vi "Pre Launch Init.vi"(11 "CameraTestingUI in":refnum<class "CameraTestingENI.lvclass">) -> (0 "error out":errorcluster, 3 "CameraTestingUI out":refnum<class "CameraTestingENI.lvclass">)   [LabVIEW 2020, in "CameraTestingProxy.lvlib" / "CameraTestingENI.lvclass"]
doc: "(<B>Filename</B>: Actor Framework.lvlib:Actor.lvclass:Pre Launch Init.vi)\n\nDefines behavior that occurs after the Launch Nested Actor method is invoked but before the actor's Actor Core method begins running.\n\nBy default, this method does nothing. A descendant class may override it to define behavior."
uses:
  CameraTestingENI.lvclass
  Private/TypeDef/PreLaunchInitState.ctl
  CameraTestingENI.lvclass/CameraTestingENI.ctl
  CameraTestingApp/ICameraTesting/ICameraTesting/TypeDef/Events.ctl
  Camera/ICamera/ICamera/TypeDef/SnapInfo.ctl
  CameraTestingApp/ICameraTesting/ICameraTesting/TypeDef/FrameRateValReceived.ctl
  CameraTestingApp/ICameraTesting/ICameraTesting/TypeDef/ImgTypeValReceived.ctl
  CameraTestingApp/ICameraTesting/ICameraTesting/TypeDef/ResolutionValReceived.ctl
  CameraTestingApp/ICameraTesting/ICameraTesting/TypeDef/VideoOptCodesUpdated.ctl
  CameraTestingApp/ICameraTesting/ICameraTesting/TypeDef/VideoOptionsInfo.ctl
  CameraTestingApp/ICameraTesting/ICameraTesting/TypeDef/StatusUpdated.ctl
  CameraTestingApp/ICameraTesting/ICameraTesting/TypeDef/StatusRecord.ctl
  CameraTestingApp/ICameraTesting/ICameraTesting/TypeDef/VideoBufferUpdate.ctl
  Private/TypeDef/CamTestEnqrReceived.ctl
  Private/TypeDef/QuitActorEvn.ctl
  Private/TypeDef/HelperLoopCamTestEvn.ctl
  Private/TypeDef/VideoLoopCamTestEvn.ctl
  <vilib>/ActorFramework/Actor/Actor.lvclass
  Camera/ICamera/ICamera/ICamera.lvclass
  CameraTestingApp/ICameraTesting/ICameraTesting/ICameraTesting.lvclass
  <vilib>/ActorFramework/Message Enqueuer/Message Enqueuer.lvclass
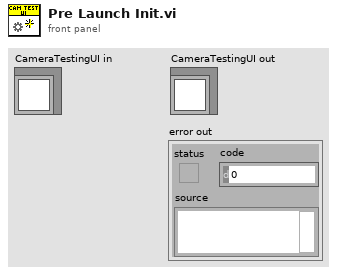
[diagram p1: front panel]
types:
  T1 = typedef "CameraTestingProxy.lvlib/CameraTestingENI.lvclass/PreLaunchInitState.ctl" = enum16{"Create Events", "Registration Events"}
  T2 = typedef "CameraTestingProxy.lvlib/CameraTestingENI.lvclass/CamTestEnqrReceived.ctl" = refnum<user-event>
  T3 = cluster{"UpdCamTestEvnReg":refnum<user-event>, "CamTestEnqrRcv":T2}
  T4 = typedef "CameraTestingProxy.lvlib/CameraTestingENI.lvclass/QuitActorEvn.ctl" = refnum<user-event>
  T5 = cluster{"UpdCamTestEvnReg":refnum<user-event>, "QuitActorFired":T4}
  T6 = typedef "CameraTestingProxy.lvlib/CameraTestingENI.lvclass/PrivateEvents.ctl" = cluster{"UpdCamTestEvnReg":refnum<user-event>, "CamTestEnqrRcv":T2, "QuitActorFired":T4}
  T7 = typedef "CameraTestingProxy.lvlib/CameraTestingENI.lvclass/RequestEventList.ctl" = cluster{"ConnectCmd":refnum<user-event>, "PlayCmd":refnum<user-event>, "SnapShoot":refnum<user-event>, "GetResolution":refnum<user-event>, "GetImageType":refnum<user-event>, "GetFrameRate":refnum<user-event>, "SetResolution":refnum<user-event>, "SetImageType":refnum<user-event>, "SetFrameRate":refnum<user-event>, "AcqVideoOptCodes":refnum<user-event>}
  T8 = typedef "CameraTestingProxy.lvlib/CameraTestingENI.lvclass/HelperLoopEvntRegRef.ctl" = refnum<event-registration>
  T9 = typedef "CameraTestingProxy.lvlib/CameraTestingENI.lvclass/VideoLoopEnvRgstRef.ctl" = refnum<event-registration>
  T10 = typedef "CameraTestingProxy.lvlib/CameraTestingENI.lvclass/VideoLoopCamTestEvn.ctl" = cluster{"VideoBufferUpdate":T11}
  T11 = typedef "ICameraTesting.lvlib/ICameraTesting.lvclass/VideoBufferUpdate.ctl" = refnum<user-event>
  T12 = typedef "CameraTestingProxy.lvlib/CameraTestingENI.lvclass/HelperLoopCamTestEvn.ctl" = cluster{"NewSnapData":refnum<user-event>, "FrameRateValReceived":T13, "ImgTypeValReceived":T14, "ResolutionValReceived":T15, "VideoOptInfoUpdated":T16, "StatusUpdated":T17}
  T13 = typedef "ICameraTesting.lvlib/ICameraTesting.lvclass/FrameRateValReceived.ctl" = refnum<user-event>
  T14 = typedef "ICameraTesting.lvlib/ICameraTesting.lvclass/ImgTypeValReceived.ctl" = refnum<user-event>
  T15 = typedef "ICameraTesting.lvlib/ICameraTesting.lvclass/ResolutionValReceived.ctl" = refnum<user-event>
  T16 = typedef "ICameraTesting.lvlib/ICameraTesting.lvclass/VideoOptCodesUpdated.ctl" = refnum<user-event>
  T17 = typedef "ICameraTesting.lvlib/ICameraTesting.lvclass/StatusUpdated.ctl" = refnum<user-event>
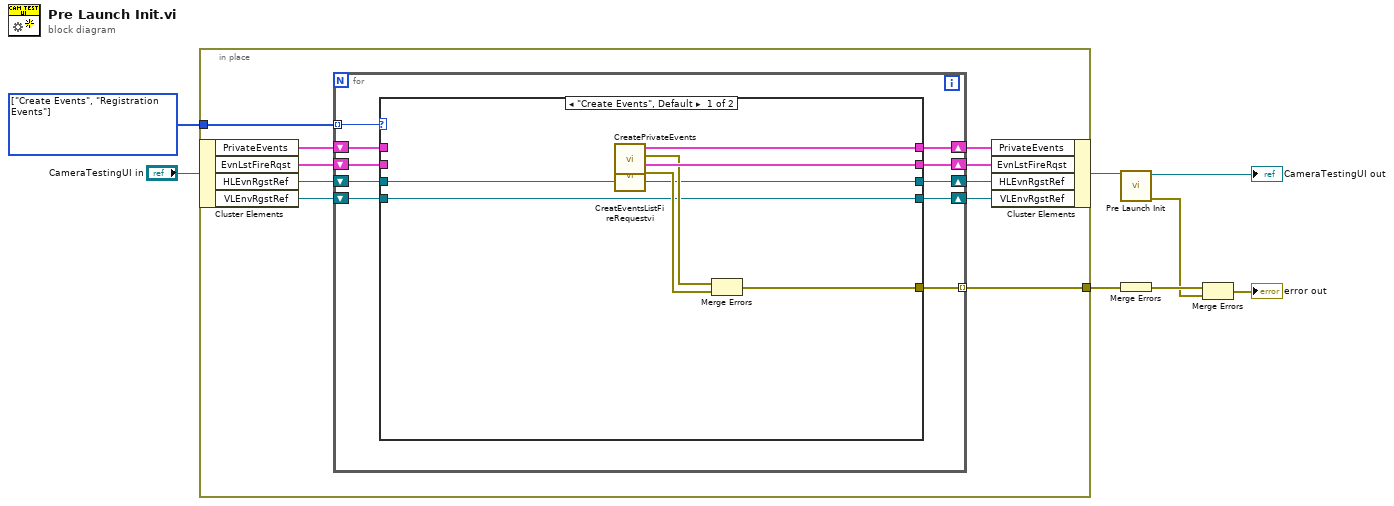
[diagram p0: block diagram]
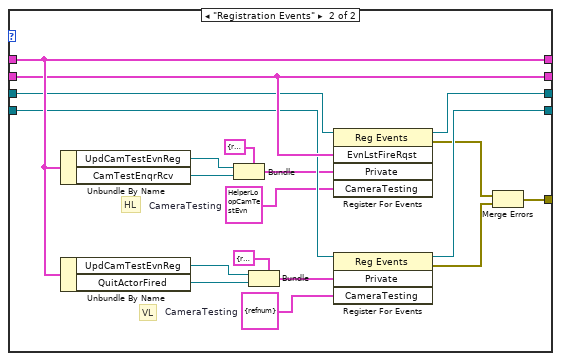
[diagram p2: hidden frame]
diagram:
  w8 = T1[] [enum."Create Events", enum."Registration Events"] items=["Create Events", "Registration Events"]
  n1 = in-place {
    in-place-border: w8 -> [w18]
    in-place-border: [w17] -> w3
    n2 = in-place-cluster #1("CameraTestingUI in") -> ("PrivateEvents"=w16:T6, "EvnLstFireRqst"=w15:T7, "HLEvnRgstRef"=w14:T8, "VLEnvRgstRef"=w13:T9)
    n3 = for {
      tunnel: [w28] -> w17 mode=indexing
      tunnel: w18 -> [w27] mode=indexing
      shift-right: [w24] -> w12
      shift-left: w16 -> [w26]
      shift-right: [w23] -> w11
      shift-left: w15 -> [w25]
      shift-right: [w21] -> w10
      shift-left: w14 -> [w22]
      shift-right: [w20] -> w9
      shift-left: w13 -> [w19]
      n4 = case shown="\"Create Events\", Default" w27 {
        tunnel: [w35 w54] -> w28
        tunnel: w26 -> [_ w53]
        tunnel: w25 -> [_ w52]
        tunnel: [w34 w53] -> w24
        tunnel: [w33 w52] -> w23
        tunnel: w22 -> [w30 w51]
        tunnel: [w30 w50] -> w21
        tunnel: [w29 w49] -> w20
        tunnel: w19 -> [w29 w48]
        frame "Create Events", Default {
          n5 = call "CreatePrivateEvents.vi"() -> ("error out"=w32:errorcluster, "PrivateEvents"=w34:T6)  [unwired: 10 in]
          n6 = call "CreatEventsListFireRequestvi.vi"() -> ("error out"=w31:errorcluster, "EvnLstFireRqst"=w33:T7)  [unwired: 10 in]
          n7 = Merge Errors(w32, w31) -> (w35:errorcluster)
        }
        frame "Registration Events" {
          w42 = T10 {"VideoBufferUpdate"=refnum}  # CameraTesting
          w37 = T12 {"NewSnapData"=refnum, "FrameRateValReceived"=refnum, "ImgTypeValReceived"=refnum, "ResolutionValReceived"=refnum, "VideoOptInfoUpdated"=refnum, "StatusUpdated"=refnum}  # CameraTesting
          # "VL"
          # "HL"
          n8 = Unbundle By Name(w53) -> ("UpdCamTestEvnReg"=w40:refnum<user-event>, "CamTestEnqrRcv"=w39:T2)
          n9 = Unbundle By Name(w53) -> ("UpdCamTestEvnReg"=w41:refnum<user-event>, "QuitActorFired"=w45:T4)
          n10 = Bundle(cluster=T3 {"UpdCamTestEvnReg"=refnum, "CamTestEnqrRcv"=refnum} ("Private"), "UpdCamTestEvnReg"=w40, "CamTestEnqrRcv"=w39) -> (w38:T3)
          n11 = Bundle(cluster=T5 {"UpdCamTestEvnReg"=refnum, "QuitActorFired"=refnum} ("Private"), "UpdCamTestEvnReg"=w41, "QuitActorFired"=w45) -> (w43:T5)
          n12 = register-events(reference=w51, w52, w38, w37) -> (reference out=w50:T8, error out=w47:errorcluster)  [unwired: 1 in]
          n13 = register-events(reference=w48, w43, w42) -> (reference out=w49:T9, error out=w46:errorcluster)  [unwired: 1 in]
          n14 = Merge Errors(w47, w46) -> (w54:errorcluster)
        }
      }
    }
    n15 = in-place-cluster #1("PrivateEvents"=w12, "EvnLstFireRqst"=w11, "HLEvnRgstRef"=w10, "VLEnvRgstRef"=w9) -> (w1:refnum<class "CameraTestingENI.lvclass">)
  }
  n16 = call-parent "Pre Launch Init.vi"("Actor in"=w1) -> ("error out"=w5:errorcluster, "Actor out"=→"CameraTestingUI out":refnum<class "CameraTestingENI.lvclass">)  [unwired: 9 in]
  n17 = Merge Errors(w3) -> (w6:errorcluster)
  n18 = Merge Errors(w6, w5) -> (→"error out":errorcluster)
